vi "EnFlo_Lab_Temp_Control.vi"() -> ()   [LabVIEW 2013]
uses:
  ADAM Client/Sub VIs/ADAM Controls/Update_scan_value.ctl
panel:
  out "EnFlo Lab:labstrat1:Av Temp":dbl
  out "EnFlo_Tunnel:Exit Duct:Dem Temp":dbl
  out "Reduction in air temp from ambient":dbl
  out "Approx Heat Extraction Value in kW":dbl
  out "EnFlo Lab:Desired:Air Temp":dbl
  out "Temperature Error":dbl
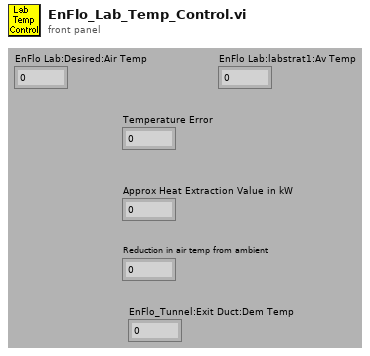
[diagram p1: front panel]
types:
  T1 = enum16{"Append to Global", "Read Global then Clear"}
  T2 = typedef "Update_scan_value.ctl" = cluster{"Channel Name":string, "New Value":dbl}
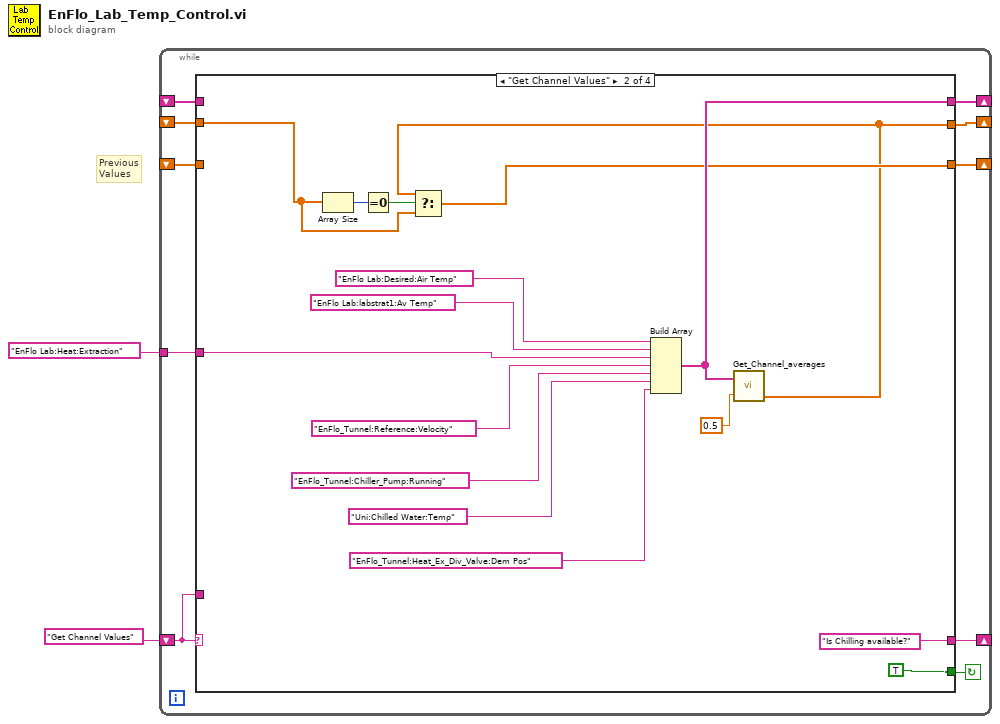
[diagram p0: block diagram]
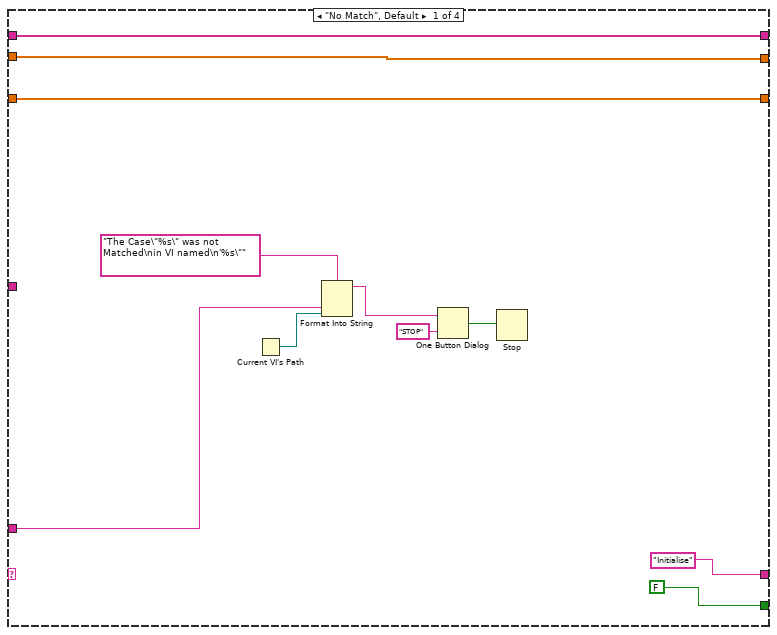
[diagram p2: hidden frame]
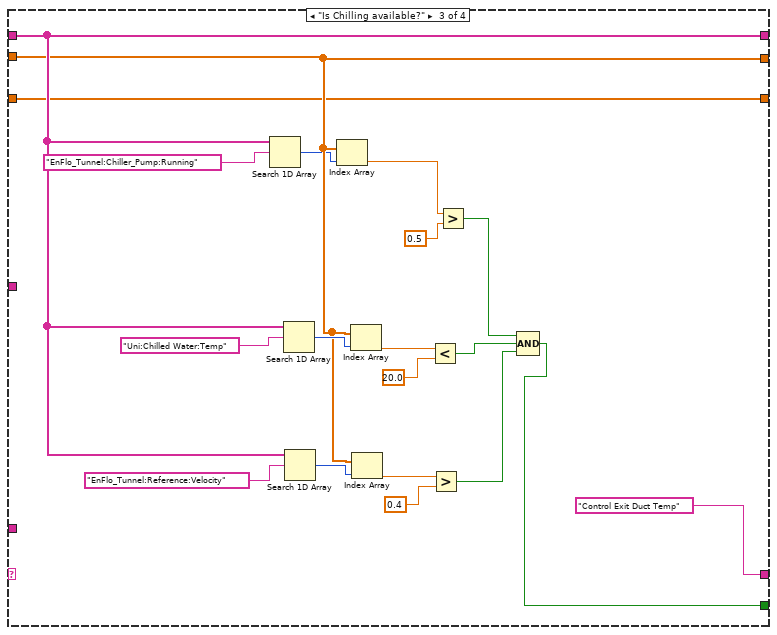
[diagram p3: hidden frame]
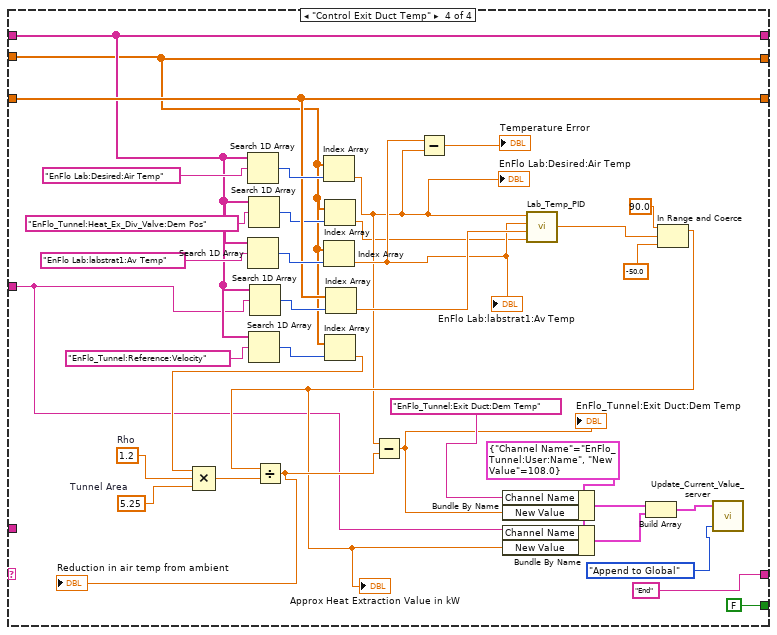
[diagram p4: hidden frame]
diagram:
  # "Previous\nValues"
  n1 = while {
    shift-left: "Get Channel Values" -> [w10]
    shift-right: [w11] -> _
    shift-right: [w8] -> _
    shift-left: _ -> [w6]
    shift-right: [w9] -> _
    shift-left: _ -> [w7]
    shift-right: [w5] -> _
    shift-left: _ -> [w4]
    tunnel: "EnFlo Lab:Heat:Extraction" -> [w3]
    stop <- w12 continue-if-true
    n2 = case shown="\"Get Channel Values\"" w10 {
      tunnel: [FALSE TRUE w40 FALSE] -> w12
      tunnel: ["Initialise" "Is Chilling available?" "Control Exit Duct Temp" "End"] -> w11
      tunnel: w10 -> [w18 _ _ _]
      tunnel: [w15 w24 w46 w62] -> w9
      tunnel: [w14 w32 w47 w64] -> w8
      tunnel: w7 -> [w15 w25 w46 w62]
      tunnel: w6 -> [w14 _ w47 w64]
      tunnel: [w13 w26 w45 w85] -> w5
      tunnel: w4 -> [w13 _ w45 w85]
      tunnel: w3 -> [_ w29 _ w60]
      frame "No Match", Default {
        n3 = Current VI's Path() -> (path=w17:path)
        n4 = Format Into String(format string="The Case\"%s\" was not Matched\nin VI named\n'%s\"" ("Format String"), w18, w17) -> (resulting string=w21:string)  [unwired: 2 in, 1 out]
        n5 = One Button Dialog(message=w21, button name ("OK")="STOP") -> (true=w19:bool)
        n6 = Stop(stop? (T)=w19) -> ()
      }
      frame "Get Channel Values" {
        n7 = Array Size(array=w25) -> (size(s)=w28:i32)
        n8 = Equal To 0?(x=w28) -> (x = 0?=w27:bool)
        n9 = Build Array("EnFlo Lab:Desired:Air Temp", "EnFlo Lab:labstrat1:Av Temp", w29, "EnFlo_Tunnel:Reference:Velocity", "EnFlo_Tunnel:Chiller_Pump:Running", "Uni:Chilled Water:Temp", "EnFlo_Tunnel:Heat_Ex_Div_Valve:Dem Pos") -> (w32:string[])
        n10 = call "Get_Channel_averages.vi"("Desired Ch Names"=w32, "Averaging time (mins)"=0.5) -> ("number"=w24:dbl[])  [unwired: 1 in, 2 out]
        n11 = Select(t=w24, s=w27, f=w25) -> (s? t:f=w26:dbl[])
      }
      frame "Is Chilling available?" {
        n12 = Search 1D Array(1D array=w47, element="EnFlo_Tunnel:Chiller_Pump:Running") -> (index of element=w44:i32)  [unwired: 1 out]
        n13 = Search 1D Array(1D array=w47, element="Uni:Chilled Water:Temp") -> (index of element=w57:i32)  [unwired: 1 out]
        n14 = Search 1D Array(1D array=w47, element="EnFlo_Tunnel:Reference:Velocity") -> (index of element=w52:i32)  [unwired: 1 out]
        n15 = Index Array(array=w46, index=w44) -> (element=w41:dbl)
        n16 = Index Array(array=w46, index=w57) -> (element=w56:dbl)
        n17 = Index Array(array=w46, index=w52) -> (element=w53:dbl)
        n18 = Less?(x=w56, y=20.0) -> (x < y?=w50:bool)
        n19 = Greater?(x=w53, y=0.4) -> (0:w49:bool)
        n20 = Greater?(x=w41, y=0.5) -> (0:w42:bool)
        n21 = Compound Arithmetic op=AND(w42, w50, w49) -> (w40:bool)
      }
      frame "Control Exit Duct Temp" {
        w70 = T2 {"Channel Name"="EnFlo_Tunnel:User:Name", "New Value"=108.0} ("Update Scan Value Cluster")
        w82 = 5.25  # Tunnel Area
        w83 = 1.2  # Rho
        n22 = Search 1D Array(1D array=w64, element="EnFlo Lab:Desired:Air Temp") -> (index of element=w95:i32)  [unwired: 1 out]
        n23 = Search 1D Array(1D array=w64, element="EnFlo Lab:labstrat1:Av Temp") -> (index of element=w91:i32)  [unwired: 1 out]
        n24 = Search 1D Array(1D array=w64, element="EnFlo_Tunnel:Heat_Ex_Div_Valve:Dem Pos") -> (index of element=w65:i32)  [unwired: 1 out]
        n25 = Search 1D Array(1D array=w64, element="EnFlo_Tunnel:Reference:Velocity") -> (index of element=w86:i32)  [unwired: 1 out]
        n26 = Search 1D Array(1D array=w64, element=w60) -> (index of element=w90:i32)  [unwired: 1 out]
        n27 = Index Array(array=w62, index=w95) -> (element=w66:dbl)
        "EnFlo Lab:Desired:Air Temp" <- w66
        n28 = Index Array(array=w62, index=w91) -> (element=w68:dbl)
        "EnFlo Lab:labstrat1:Av Temp" <- w68
        n29 = Index Array(array=w62, index=w65) -> (element=w61:dbl)
        n30 = Index Array(array=w62, index=w86) -> (element=w84:dbl)
        n31 = Compound Arithmetic op=MULTIPLY(w84, w83, w82) -> (w81:dbl)
        n32 = Index Array(array=w85, index=w90) -> (element=w89:dbl)
        n33 = Subtract(x=w68, y=w66) -> (x-y=→"Temperature Error":dbl)
        n34 = call "Lab_Temp_PID.vi"("Valve Pos"=w61, "Previous Control Sum"=w89, "Present Value"=w68, "Setpoint"=w66) -> ("Dem Output"=w69:dbl)
        n35 = In Range and Coerce(upper limit=90.0, x=w69, lower limit=-50.0) -> (coerced(x)=w72:dbl)  [unwired: 1 out]
        "Approx Heat Extraction Value in kW" <- w72
        n36 = Divide(x=w72, y=w81) -> (x/y=w80:dbl)
        "Reduction in air temp from ambient" <- w80
        n37 = Subtract(x=w66, y=w80) -> (x-y=w76:dbl)
        "EnFlo_Tunnel:Exit Duct:Dem Temp" <- w76
        n38 = Bundle By Name(cluster=w70, "Channel Name"="EnFlo_Tunnel:Exit Duct:Dem Temp", "New Value"=w76) -> (w73:T2)
        n39 = Bundle By Name(cluster=w70, "Channel Name"=w60, "New Value"=w72) -> (w71:T2)
        n40 = Build Array(w73, w71) -> (w78:T2[])
        n41 = call "Update_Current_Value_server.vi"("Mode"=T1."Append to Global", "Update array in"=w78) -> ()  [unwired: 1 in, 1 out]
      }
    }
  }
